vi "LabVIEW_MQTT_Toolkit_V2.vi"() -> ()   [LabVIEW 2021]
uses:
  class/mqtt/mqttTypedef/mqttQOSlevel.ctl
  class/mqtt/mqttTypedef/mqttConnectionStatus.ctl
  class/mqtt/mqttTypedef/mqttBroker.ctl
  class/mqtt/mqttTXqueue/mqttTXdataQueueFunction.ctl
  class/mqtt/mqttConfigFunction.ctl
  class/mqtt/mqttTXqueue/mqttRXsubscriptionEventFunction.ctl
  <vilib>/Utility/sysdir.llb/System Directory Type.ctl
  library/Epoch Date & Time/epoch.UNIX/Epoch.UNIX.lvclass
  C:/Users/Fujitsu/Desktop/labpublish/avril/Project mqtt/Src/library/Epoch Date & Time/epoch/Epoch.lvclass
  <vilib>/Utility/file.llb/Write Delimited Spreadsheet (string).vi
  library/Epoch Date & Time/Get Epoch Time.vi
  class/mqtt/mqtt.lvclass
panel:
  out "concatenated string":string
  in  "Tab Control":T1(tab)
  in  "Device type":u16(ring) items=["AX_3D", "AX_3DS", "HI_INC_BI", "HI_INC_MONO", "X_INC_BI", "X_INC_MONO"]
  in  "Tx ratio":u8
  in  "Store and forward":bool
  in  "Streaming options":T2(radio)
  in  "Daq options":T3(radio)=enum."Tx Only"
  out "Connection Success":bool
  in  "connect":bool
  out "ConnStatus":T4
  in  "disconnect":bool
  in  "subscribe":bool
  out "Subscribe Success":bool
  in  "Subscription_Info":cluster{"Topic":string, "QoS":T5}[](array[cluster])=[{"Topic"="MacID/Topic", "QoS"=enum."At most once"}]
  out "Subscribed_Topic":string
  out "messageID":u16
  in  "quit":bool
  in  "Broker configuration":T6={"IP or  URL of the broker"="", "connTimeout"=2000, "writeTimeout"=2000, "readTimeout"=2000, "subTimeout"=30000, "Port"=1883}
  in  "Topic":string
  out "Publish success":bool
  in  "Publish":bool
  in  "Data acq .mode":u8(ring)=1 items=["Stop"=1, "LowDutyCycle"=2, "Alarm"=4, "Streaming"=3, "S.E.T"=5, "Sock Detection"=6]
  in  "Data Acq duration":cluster{"hours":u8, "minutes":u8, " Seconds":u8} {"Seconds" max=60 format="%02.0f"; "minutes" max=60 format="%02.0f"; "hours" max=24 format="%02.0f"}
  in  "Sampling rate":u32(ring) items=["", "10 Hz", "16 Hz", "20 Hz", "25 Hz", "32 Hz", "40 Hz", "50 Hz", "64 Hz", "80 Hz", "100 Hz", "125 Hz", "160 Hz", "200 Hz", "250  Hz", "320 Hz", "400 Hz", "500 Hz", "800 Hz", "1000 Hz", "1600 Hz", "2000 Hz"]
  in  "Data acq cycle/Notif cycle":cluster{"hours":u8, "minutes":u8, " Seconds":u8} {"Seconds" max=60 format="%02.0f"; "minutes" max=60 format="%02.0f"; "hours" max=24 format="%02.0f"}
  in  "Data aging":u16=30 step=10
  in  "Mac Id":string
  in  "Math notif ratio":u16
  in  "Ping request":bool
  out "Measure Graph":dbl(graph)
  out "Measure mode":string
  out "Sensor Label":string
  out "Measure":dbl
  out "Date & time":string
  out "Device type":string
  out "End date":string
  out "Start date":string
  out "Average value":dbl
  out "Minimum value":dbl
  out "Maximum value":dbl
  out "Date":string
  out "Date":string
  out "File path":path
  out "File path":path
  out "Measure mode":string
  out "Sensor label":string
  out "Measure":dbl
  out "Date & time":string
  out "Device type":string
  out "Alarm status":string
  out "Waveform Chart":dbl(graph) caption="Measure graph"
  out "File path":path
  out "Sampling rate":i16
  out "Frame sequence Id":u32
  out "Number of daq per channel":u16
  out "Data acquisition cycle":u32
  out "Data acquisition duration":u32
  out "Prev.number of daq per channel":u16
  out "Enabled channels":string
  out "Device type":string
  out "Measure mode":string
  out "millisec":u16
  out "not synchronised":bool
  out "synchronised":bool
  out "Network quality (LQI)":u8 format="%.0p"
  out "Ref time":string
  out "INC_Y Graph":dbl[](graph)
  out "CH_Z Graph":dbl[](graph)
  out "CH_X Graph":dbl[](graph)
  out "CH_Y Graph":dbl[](graph)
  out "INC_X Graph":dbl[](graph)
  out "File path":path
  out "Enabled channels":string
  out "Device type":string
  out "Measure mode":string
  out "Frame sequence Id":u32
  out "Number of daq per channel":u16
  out "Data notification cycle":u32
  out "Data acquisition duration":u32
  out "Prev.number of daq per channel":u16
  out "not synchronised":bool
  out "synchronised":bool
  out "Network quality (LQI)":u8 format="%.0p"
  out "Sampling rate":i16
  out "millisec":u16
  out "Ref time":string
  out "channel that received alarm":u8
  out "CH_Z Graph":dbl[](graph)=[0.984, 0.974, 0.974, 0.986, 1.009, 0.965, 0.949, 0.987, 0.909, 0.979, 0.976, 1.021, 0.92, 0.95, 1.042, 0.989, 0.939, 1.09, 0.874, 0.972, 0.98, 0.977, 0.963, 0.971, 0.982, 0.977, 0.992, 0.993, 0.98, 0.969, 0.975, 0.969, 0.986, 0.985, 0.978, 0.977, 0.982, 0.979, 0.977, 0.972, 0.967, 0.968, 0.986, 0.97, 0.973, 0.977, 0.982, 0.973, 0.953, 0.969, 0.983, 0.968, 0.965, 0.975, 0.974, 0.972, 0.983, 0.99, 0.968, 0.972, 0.97, 0.981, 0.968, 0.982, 0.979, 0.972]
  out "CH_X Graph":dbl[](graph)=[0.011, 0.001, 0.002, 0.005, 0.007, 0.003, 0.001, 0.011, -0.001, 0.008, 0.006, 0.001, -0.001, 0.017, -0.002, 0.004, 0.0, -0.007, 0.002, -0.007, 0.001, 0.002, 0.0, 0.003, 0.004, 0.009, 0.004, 0.012, 0.003, 0.003, 0.004, 0.003, 0.006, 0.001, -0.001, 0.003, 0.002, 0.001, 0.003, 0.0, -0.001, 0.005, 0.0, 0.005, 0.001, 0.005, 0.005, -0.001, -0.002, -0.001, 0.005, 0.003, -0.003, -0.003, 0.002, -0.002, 0.002, 0.007, 0.0, 0.0, -0.002, 0.001, 0.002, 0.005, 0.011, 0.006]
  out "CH_Y Graph":dbl[](graph)=[-0.006, -0.012, -0.012, -0.009, -0.015, 0.009, 0.007, -0.013, 0.026, 0.009, -0.014, -0.014, 0.046, 0.055, -0.014, 0.004, 0.027, -0.027, 0.076, -0.008, -0.016, -0.026, -0.02, -0.015, -0.01, -0.002, -0.005, -0.011, -0.019, -0.019, -0.014, -0.009, -0.01, -0.01, -0.017, -0.015, -0.01, -0.013, -0.014, -0.014, -0.014, -0.014, -0.013, -0.017, -0.015, -0.013, -0.008, -0.015, -0.02, -0.017, -0.011, -0.014, -0.015, -0.016, -0.019, -0.016, -0.016, -0.012, -0.016, -0.016, -0.01, -0.013, -0.013, -0.019, -0.015, -0.012]
  out "INC_X Graph":dbl[](graph)=[0.03, 0.047, 0.036, 0.04, 0.082, 0.015, 0.021, 0.002, -0.032, 0.039, 0.026, 0.014, 0.037, 0.052, 0.099, 0.049, 0.039, 0.13, -0.382, 0.13, 0.113, 0.024, 0.006, -0.008, 0.051, 0.01, 0.082, 0.011, 0.03, 0.0, 0.031, 0.032, 0.033, 0.046, 0.032, 0.037, 0.018, 0.028, 0.024, 0.031, -0.008, 0.054, 0.011, 0.025, 0.04, 0.026, 0.022, 0.017, 0.028, 0.042, 0.024, 0.016, 0.034, 0.035, 0.018, 0.043, 0.014, 0.039, 0.033, 0.018, 0.035, 0.027, 0.041, 0.031, 0.035, 0.03]
  out "INC_Y Graph":dbl[](graph)=[0.458, 0.458, 0.458, 0.458, 0.458, 0.458, 0.458, 0.458, 0.458, 0.458, 0.458, 0.458, 0.458, 0.458, 0.458, 0.458, 0.458, 0.458, 0.458, 0.458, 0.458, 0.458, 0.458, 0.458, 0.458, 0.458, 0.458, 0.458, 0.458, 0.458, 0.458, 0.458, 0.458, 0.458, 0.458, 0.458, 0.458, 0.458, 0.458, 0.458, 0.458, 0.458, 0.458, 0.458, 0.458, 0.458, 0.458, 0.458, 0.458, 0.458, 0.458, 0.458, 0.458, 0.458, 0.458, 0.458, 0.458, 0.458, 0.458, 0.458, 0.458, 0.458, 0.458, 0.458, 0.458, 0.458]
  out "File path":path
  out "File path":path
  out "Data acquisition duration":u32
  out "Frame sequence Id":u32
  out "Data monitoring cycle":u32
  out "Device type":string
  out "Sampling rate":i16
  out "Number of daq per channel":u16
  out "Prev.number of daq per channel":u16
  out "Ref time":string
  out "millisec":u16
  out "Measure mode":string
  out "Enabled channels":string
  out "Network quality (LQI)":u8 format="%.0p"
  out "CH_Z Graph":dbl[](graph)
  out "synchronised":bool
  out "not synchronised":bool
  out "CH_Y Graph":dbl[](graph)
  out "CH_X Graph":dbl[](graph)
  out "Shock source":string
  out "Y Axis first data":dbl format="%#_5f"
  out "X Axis first data":dbl format="%#_5f"
  out "Z Axis first data":dbl format="%#_5f"
  out "Device type":string
  out "Acquisition Mode":string
  out "Acquisition frequency":u16
  out "Acquisition cycle":u32
  out "Acquisition duration":u32
  out "Enabled channels":string
  out "Start date":string
  out "End date":string
  out "Number of data per channel":u16
  out "fid min ch1":u32
  out "index minval":u16
  out "fid max ch1":u32
  out "index maxval":u16
  out "Max value":dbl[](array[numeric]) format="%#_3g"
  out "Average value":dbl[](array[numeric])
  out "Min value":dbl[](array[numeric])
  out "String":string="Ch_Z                    Ch_X                     Ch_Y                     INC_X                     INC_Y"
  out "File path":path
  out "Min date":string[](array[string])
  out "Max date":string[](array[string])
  out "Numeric":i32
  # "Publish_Info"
  # ":"
  # ":"
  # "HH:MM:SS"
  # ":"
  # ":"
  # "HH:MM:SS"
  # "LowDutyCycle Measurement"
  # "MathMode Result"
  # "AlarmMode Measurement"
  # "StreamingMode Measurement"
  # "S.E.T Mode Measurement"
  # "ShockDetectionMode Measurement"
  # "DynamicMathMode Measurement"
types:
  T1 = enum32{"Configuration", "LowDutyCycleData", "AlarmData ", "StreamingModeData", "S.E.T Mode", "Shock Detection", "Dynamic Math Result"}
  T2 = enum32{"No Selection", "Continuous Monitoring", "Burst", "One Shot"}
  T3 = enum32{"No Selection", "Tx Only", "Log Only", "Tx&Log", "SA"}
  T4 = typedef "mqttConnectionStatus.ctl" = enum16{"Connection accepted", "Connection refused: unacceptable protocol version", "Connection refused: identifier rejected", "Connection refused: Server unavailable", "Connection refused: bad user name or password", "Connection refused: not authorized"}
  T5 = typedef "mqttQOSlevel.ctl" = enum8{"At most once", "At least once", "Exactly once", "Reserved"}
  T6 = typedef "mqttBroker.ctl" = cluster{"IP or  URL of the broker":string, "connTimeout":i32, "writeTimeout":i32, "readTimeout":i32, "subTimeout":i32, "Port":u16}
  T7 = typedef "mqttRXsubscriptionEventFunction.ctl" = enum16{"init", "deinit", "getEventRef", "event"}
  T8 = typedef "mqtt.lvclass/mqttConfigFunction.ctl" = enum16{"init", "deinit", "set", "get"}
  T9 = typedef "mqttTXdataQueueFunction.ctl" = enum16{"init", "deinit", "getQueue", "enqueue"}
  T10 = enum8{"Enabled", "Disabled", "Disabled and Grayed Out"}
  T11 = enum16{"open", "replace", "create", "open or create", "replace or create", "replace or create with confirmation"}
  T12 = cluster{"[0]":u8, "[1]":u8, "[2]":u8, "[3]":u8, "[4]":u8, "[5]":u8, "[6]":u8, "[7]":u8, "[8]":u8}
  T13 = cluster{"[0]":u8, "[1]":u8, "[2]":u8, "[3]":u8, "[4]":u8, "[5]":u8, "[6]":u8, "[7]":u8, "[8]":u8, "[9]":u8, "[10]":u8, "[11]":u8, "[12]":u8}
  T14 = typedef "System Directory Type.ctl" = i32
  T15 = cluster{"unsigned byte array[0]":u8, "unsigned byte array[1]":u8}
  T16 = cluster{"[0]":u8, "[1]":u8, "[2]":u8, "[3]":u8, "[4]":u8, "[5]":u8, "[6]":u8, "[7]":u8, "[8]":u8, "[9]":u8, "[10]":u8, "[11]":u8, "[12]":u8, "[13]":u8, "[14]":u8, "[15]":u8}
  T17 = cluster{"[0]":u8, "[1]":u8, "[2]":u8, "[3]":u8, "[4]":u8, "[5]":u8, "[6]":u8, "[7]":u8, "[8]":u8, "[9]":u8, "[10]":u8, "[11]":u8, "[12]":u8, "[13]":u8, "[14]":u8, "[15]":u8, "[16]":u8, "[17]":u8, "[18]":u8, "[19]":u8, "[20]":u8, "[21]":u8}
  T18 = cluster{"unsigned byte array[0]":u8, "unsigned byte array[1]":u8, "unsigned byte array[2]":u8, "unsigned byte array[3]":u8, "unsigned byte array[4]":u8, "unsigned byte array[5]":u8, "unsigned byte array[6]":u8, "unsigned byte array[7]":u8, "unsigned byte array[8]":u8, "unsigned byte array[9]":u8, "unsigned byte array[10]":u8, "unsigned byte array[11]":u8, "unsigned byte array[12]":u8, "unsigned byte array[13]":u8, "unsigned byte array[14]":u8, "unsigned byte array[15]":u8, "unsigned byte array[16]":u8, "unsigned byte array[17]":u8, "unsigned byte array[18]":u8, "unsigned byte array[19]":u8, "unsigned byte array[20]":u8, "unsigned byte array[21]":u8, "unsigned byte array[22]":u8, "unsigned byte array[23]":u8, "unsigned byte array[24]":u8, "unsigned byte array[25]":u8, "unsigned byte array[26]":u8, "unsigned byte array[27]":u8, "unsigned byte array[28]":u8, "unsigned byte array[29]":u8, "unsigned byte array[30]":u8, "unsigned byte array[31]":u8, "unsigned byte array[32]":u8, "unsigned byte array[33]":u8, "unsigned byte array[34]":u8, "unsigned byte array[35]":u8}
  T19 = cluster{"[0]":string, "[1]":string, "[2]":string, "[3]":string, "[4]":string}
  T20 = cluster{"[0]":dbl, "[1]":dbl, "[2]":dbl, "[3]":dbl, "[4]":dbl}
diagram:
  # "here you will find different modes of  data acquisition"
  # "cluster contain broker configuration"
  n1 = flat-sequence {
    tunnel: [w20] -> w14
    tunnel: [w17] -> w9
    frame #0 {
      w16 = T10."Disabled and Grayed Out" ("Disabled")
      n2 = property on="disconnect" class="Bool"("DisabledEnum"=w16) -> ()  [unwired: 2 in, 2 out]
      n3 = property on="subscribe" class="Bool"("DisabledEnum"=w16) -> ()  [unwired: 2 in, 2 out]
      n4 = call "mqttRXsubscriptionEvent.vi"("function"=mqttRXsubscriptionEventFunction."init") -> ("subscriptionData"=w17:refnum<user-event>, "error out"=w19:errorcluster)  [unwired: 13 in]
      n5 = call "mqttTXdataQueue.vi"("function"=mqttTXdataQueueFunction."init", "error in (no error)"=w19) -> ("error out"=w20:errorcluster)  [unwired: 12 in, 1 out]
    }
  }
  n6 = register-events(w9) -> (reference out=w8:refnum<event-registration>)  [unwired: 2 in, 1 out]
  n7 = call "api_mqttInit.vi"("broker"="Broker configuration", "error in (no error)"=w14) -> ("error out"=w12:errorcluster)  [unwired: 13 in]
  n8 = call "mqttConfigStore.vi"("function"=mqttConfigFunction."get", "error in (no error)"=w12) -> ("mqtt.lvclass out"=w11:refnum<class "mqtt.lvclass">, "error out"=w1:errorcluster)  [unwired: 12 in]
  n9 = call "mqttTCPIPserver.vi"("mqtt.lvclass"=w11, "error in (no error)"=w1) -> ()  [unwired: 12 in, 2 out]
  n10 = while {
    shift-right: [w27] -> w5
    shift-left: w1 -> [w22]
    tunnel: w8 -> [w26]
    tunnel: [w25] -> w3
    i -> [w23]
    stop <- w24 stop-if-true
    n11 = event shown="[5] \"subscribe\": Value Change" {
      selector: w26 -> [_ _ _ _ _ _ _ _ _ _ _]
      dyn-events: [_ _ _ _ _ _ _ _ _ _ _] -> w25
      timeout: _ -> [_ _ _ _ _ _ _ _ _ _ _]
      tunnel: [w31 w115 w159 w162 w165 w169 w254 w6078 w6108 w6119 w6128] -> w27
      tunnel: w22 -> [w31 w116 w159 w163 w166 w167 w254 w6078 w6108 w6119 w6128]
      tunnel: [TRUE _ _ _ _ _ _ _ _ _ _] -> w24
      tunnel: w23 -> [_ _ _ _ _ _ w175 _ _ _ _]
      event "quit": Value Change {
        # "used to reinitialize to default  data when you execute VI"
        # "when we press quit in front panel the process is stopped"
        n12 = event-data() -> ()  [unwired: 1 in, 1 out]
        n13 = control-ref of="This VI"() -> (w30:refnum<vi>)
        n14 = invoke class="VI" method="Default Vals.Reinit All"(reference=w30) -> (reference out=w28:refnum<vi>, error out=w29:errorcluster)  [unwired: 2 in, 1 out]
        n15 = Close Reference(reference=w28, error in (no error)=w29) -> ()  [unwired: 1 out]
      }
      event "Publish": Value Change {
        w37 = u8 0
        w38 = u8 0
        w52 = u8 16
        w53 = u8 23
        # "publish button"
        # "this is math constant \"3600\" to stop the process"
        n16 = event-data() -> ()  [unwired: 1 in, 1 out]
        n17 = String Subset(string="Mac Id", length (rest)=15 ("length (rest)")) -> (substring=w112:string)  [unwired: 1 in]
        n18 = String Length(string=w112) -> (length=w113:i32)
        n19 = call <vilib>:"Trim Whitespace.vi"("string"=w112) -> ("trimmed string"=w111:string)  [unwired: 1 in]
        n20 = for {
          N: w113 -> [_]
          tunnel: w111 -> [w158]
          tunnel: [w155] -> w110 mode=indexing
          i -> [w154]
          n21 = Multiply(x=w154, y=2) -> (x*y=w152:i32)
          n22 = String Subset(string=w158, offset (0)=w152, length (rest)=2 ("length (rest)")) -> (substring=w156:string)
          n23 = Hexadecimal String To Number(string=w156) -> (number=w155:u32)  [unwired: 2 in, 1 out]
        }
        n24 = Unbundle By Name("Data acq cycle/Notif cycle") -> ("hours"=w85:u8, "minutes"=w84:u8, "Seconds"=w83:u8)
        n25 = Unbundle By Name("Data Acq duration") -> ("hours"=w74:u8, "minutes"=w73:u8, "Seconds"=w72:u8)
        n26 = Multiply(x=w83, y=1.0) -> (x*y=w92:dbl)
        n27 = Multiply(x=w72, y=1.0) -> (x*y=w79:dbl)
        n28 = Multiply(x=w84, y=60.0) -> (x*y=w91:dbl)
        n29 = Multiply(x=w73, y=60.0) -> (x*y=w78:dbl)
        n30 = Multiply(x=w85, y=3600.0) -> (x*y=w90:dbl)
        n31 = case shown="0, Default" "Sampling rate" {
          tunnel: [10 16 20 25 32 40 50 64 80 100 125 160 200 250 320 400 500 800 1000 1600 0 2000] -> w39
          frame 1 {
          }
          frame 2 {
          }
          frame 3 {
          }
          frame 4 {
          }
          frame 5 {
          }
          frame 6 {
          }
          frame 7 {
          }
          frame 8 {
          }
          frame 9 {
          }
          frame 10 {
          }
          frame 11 {
          }
          frame 12 {
          }
          frame 13 {
          }
          frame 14 {
          }
          frame 15 {
          }
          frame 16 {
          }
          frame 17 {
          }
          frame 18 {
          }
          frame 19 {
          }
          frame 20 {
          }
          frame 0, Default {
          }
          frame 21 {
          }
        }
        n32 = property on="Streaming options" class="RadioBtnsControl (strict)"() -> ("Value"=w44:T2)  [unwired: 2 in, 2 out]
        n33 = Add(x=w92, y=w91) -> (x+y=w89:dbl)
        n34 = Add(x=w79, y=w78) -> (x+y=w76:dbl)
        n35 = Multiply(x=w74, y=3600.0) -> (x*y=w77:dbl)
        n36 = case shown="True" "Store and forward" {
          tunnel: [u16 0 "Data aging"] -> w59
          frame False {
          }
          frame True {
          }
        }
        n37 = Add(x=w89, y=w90) -> (x+y=w71:dbl)
        n38 = Add(x=w76, y=w77) -> (x+y=w68:dbl)
        n39 = case shown="\"Tx Only\"" "Daq options" {
          tunnel: [u8 32 u8 1 u8 0 u8 33 u8 64] -> w106
          frame "Tx Only" {
          }
          frame "Log Only" {
          }
          frame "No Selection", Default {
          }
          frame "Tx&Log" {
          }
          frame "SA" {
          }
        }
        n40 = case shown="\"Continuous Monitoring\"" w44 {
          tunnel: [u8 0 ("index") u8 4 u8 12 u8 8] -> w105
          frame "No Selection", Default {
          }
          frame "Continuous Monitoring" {
          }
          frame "Burst" {
          }
          frame "One Shot" {
          }
        }
        n41 = To Unsigned Long Integer(number=w71) -> (unsigned 32bit integer=w102:u32)
        n42 = To Unsigned Long Integer(number=w68) -> (unsigned 32bit integer=w70:u32)
        n43 = To Unsigned Byte Integer(number=w110) -> (unsigned 8bit integer=w88:u8[])
        n44 = Split Number(x=w39) -> (hi(x)=w63:u16, lo(x)=w62:u16)
        n45 = Split Number(x=w102) -> (hi(x)=w100:u16, lo(x)=w101:u16)
        n46 = Split Number(x=w70) -> (hi(x)=w69:u16, lo(x)=w67:u16)
        n47 = Add(x=w106, y=w105) -> (x+y=w51:u8)
        n48 = Split Number(x=w63) -> (lo(x)=w60:u8)  [unwired: 1 out]
        n49 = Split Number(x=w100) -> (lo(x)=w96:u8)  [unwired: 1 out]
        n50 = Split Number(x=w69) -> (lo(x)=w64:u8)  [unwired: 1 out]
        n51 = Split Number(x=w62) -> (hi(x)=w56:u8, lo(x)=w61:u8)
        n52 = Split Number(x=w59) -> (hi(x)=w57:u8, lo(x)=w58:u8)
        n53 = Split Number(x="Math notif ratio") -> (hi(x)=w35:u8, lo(x)=w34:u8)
        n54 = Split Number(x=w101) -> (hi(x)=w97:u8, lo(x)=w98:u8)
        n55 = Split Number(x=w67) -> (hi(x)=w65:u8, lo(x)=w66:u8)
        n56 = Array Subset(array=w88, index=0, length=8) -> (w54:u8[])
        n57 = Build Array (concatenate)(w54, w53, w52, "Data acq .mode", w51, u8 0, u8 0, u8 0, w98, w97, w96, "Tx ratio", w66, w65, w64, w61, w56, w60, w38, w38, w38, w58, w57, w34, w35) -> (w46:u8[])
        n58 = Build Array (concatenate)(w54, w53, w52, "Data acq .mode", w51, w37, w37, w37, w37, w37, w37, "Tx ratio", w37, w37, w37, w37, w37, w37, w37, w37, w37, w37, w37, u8 16, u8 14) -> (w47:u8[])
        n59 = Equal?(x="Data acq .mode", y=u8 1) -> (x = y?=w48:bool)
        n60 = Select(t=w47, s=w48, f=w46) -> (s? t:f=w45:u8[])
        n61 = call "api_mqttPublish.vi"("topic"="Topic", "value"=w45, "QoS (At most once)"=mqttQOSlevel."At most once", "error in (no error)"=w116) -> ("success"=→"Publish success":bool, "error out"=w115:errorcluster)  [unwired: 10 in]
      }
      event "Ping request": Value Change {
        n62 = event-data() -> ()  [unwired: 1 in, 1 out]
        n63 = call "api_mqttPing.vi"("error in (no error)"=w159) -> ()  [unwired: 13 in, 2 out]
      }
      event "connect": Value Change {
        # "when the connection is accepted subscribe+disconnect become enabled"
        # "this button is to conect to the broker"
        n64 = event-data() -> ()  [unwired: 1 in, 4 out]
        n65 = call "api_mqttConnect.vi"("error in (no error)"=w163) -> ("success"=→"Connection Success":bool, "connStatus"=w161:T4, "error out"=w162:errorcluster)  [unwired: 11 in, 1 out]
        "ConnStatus" <- w161
        n66 = case shown="\"Connection accepted\"" w161 {
          frame "Connection accepted" {
            w164 = T10."Enabled" ("Disabled")
            n67 = property on="disconnect" class="Bool"("DisabledEnum"=w164) -> ()  [unwired: 2 in, 2 out]
            n68 = property on="subscribe" class="Bool"("DisabledEnum"=w164) -> ()  [unwired: 2 in, 2 out]
          }
          frame Default {
          }
        }
      }
      event "disconnect": Value Change {
        n69 = event-data() -> ()  [unwired: 1 in, 4 out]
        n70 = call "api_mqttDisconnect.vi"("error in (no error)"=w166) -> ("error out"=w165:errorcluster)  [unwired: 13 in, 1 out]
      }
      event "subscribe": Value Change {
        # "contain topic to which we will subscribe"
        # "this indicator turn to green when the subscription sucssed"
        n71 = event-data() -> ()  [unwired: 1 in, 4 out]
        n72 = feedback #1(u16 0) -> (w172:u16)
        n73 = Increment(x=w172) -> (x+1=w168:u16)
        n74 = feedback-in #1(w168) -> ()
        n75 = call "api_mqttSubscribe.vi"("subscriptionInfo"="Subscription_Info", "messageID"=w168, "error in (no error)"=w167) -> ("success"=→"Subscribe Success":bool, "error out"=w169:errorcluster)  [unwired: 11 in]
      }
      event User Event {
        n76 = event-data() -> ("topic"=w174:string, "value"=w188:string, "messageID"=→"messageID":u16)  [unwired: 1 in]
        "Subscribed_Topic" <- w174
        n77 = String To Byte Array(string=w188) -> (unsigned byte array=w196:u8[])
        n78 = Reverse 1D Array(array=w196) -> (reversed array=w240:u8[])
        n79 = Array Subset(array=w196, index=0, length=7) -> (w191:u8[])
        n80 = Array Subset(array=w196, index=7, length=1) -> (w198:u8[])
        n81 = Array Subset(array=w196, index=3, length=13) -> (w233:u8[])
        n82 = Array To Cluster(array=w191) -> (cluster=w246:T12)
        n83 = Array To Cluster(array=w198) -> (cluster=w197:cluster{"[0]":u8})
        n84 = Array To Cluster(array=w233) -> (cluster=w232:T13)
        n85 = Array Subset(array=w240, index=0, length=3) -> (w179:u8[])
        n86 = Unbundle By Name(w197) -> ("[0]"=w177:u8)
        n87 = Unbundle By Name(w232) -> ("[0]"=w189:u8, "[1]"=w212:u8, "[2]"=w211:u8, "[3]"=w210:u8, "[4]"=w209:u8, "[5]"=w216:u8, "[6]"=w215:u8, "[7]"=w214:u8, "[8]"=w213:u8, "[9]"=w206:u8, "[10]"=w205:u8, "[11]"=w208:u8, "[12]"=w207:u8)
        n88 = Unbundle By Name(w246) -> ("[0]"=w178:u8, "[1]"=w204:u8, "[2]"=w241:u8, "[3]"=w245:u8, "[4]"=w244:u8, "[5]"=w243:u8, "[6]"=w242:u8)
        n89 = Array To Cluster(array=w179) -> (cluster=w186:cluster{"[0]":u8, "[1]":u8, "[2]":u8})
        n90 = Join Numbers(hi=w244, lo=w245) -> ((hi.lo)=w236:u16)
        n91 = Join Numbers(hi=w242, lo=w243) -> ((hi.lo)=w237:u16)
        n92 = Join Numbers(hi=w211, lo=w212) -> ((hi.lo)=w227:u16)
        n93 = Join Numbers(hi=w209, lo=w210) -> ((hi.lo)=w228:u16)
        n94 = Join Numbers(hi=w215, lo=w216) -> ((hi.lo)=w222:u16)
        n95 = Join Numbers(hi=w213, lo=w214) -> ((hi.lo)=w223:u16)
        n96 = Join Numbers(hi=w205, lo=w206) -> ((hi.lo)=w217:u16)
        n97 = Join Numbers(hi=w207, lo=w208) -> ((hi.lo)=w218:u16)
        n98 = case shown="1" w178 {
          tunnel: ["AX-3D" "HI_INC_MONO" "HI_INC_BI" "X_INC_MONO " "X _INC_BI " "AX_3DS" ""] -> w187
          frame 1 {
          }
          frame 2 {
          }
          frame 3 {
          }
          frame 4 {
          }
          frame 5 {
          }
          frame 6 {
          }
          frame Default {
          }
        }
        "Device type" <- w187
        n99 = case shown="1" w241 {
          tunnel: ["Ch_Z" "Ch_Y" "INC_X" "INC_Y" "" "Ch_X"] -> w176
          frame 0 {
          }
          frame 2 {
          }
          frame 3 {
          }
          frame 4 {
          }
          frame Default {
          }
          frame 1 {
          }
        }
        n100 = Unbundle(w186) -> ("[0]"=w183:u8, "[1]"=w184:u8, "[2]"=w185:u8)
        n101 = Join Numbers(hi=w184, lo=w185) -> ((hi.lo)=w181:u16)
        n102 = To Unsigned Word Integer(number=w236) -> (unsigned 16bit integer=w249:u16)
        n103 = To Unsigned Word Integer(number=w237) -> (unsigned 16bit integer=w250:u16)
        n104 = To Unsigned Word Integer(number=w227) -> (unsigned 16bit integer=w229:u16)
        n105 = To Unsigned Word Integer(number=w228) -> (unsigned 16bit integer=w230:u16)
        n106 = To Unsigned Word Integer(number=w222) -> (unsigned 16bit integer=w224:u16)
        n107 = To Unsigned Word Integer(number=w223) -> (unsigned 16bit integer=w225:u16)
        n108 = To Unsigned Word Integer(number=w217) -> (unsigned 16bit integer=w219:u16)
        n109 = To Unsigned Word Integer(number=w218) -> (unsigned 16bit integer=w220:u16)
        n110 = Join Numbers(hi=w250, lo=w249) -> ((hi.lo)=w251:u32)
        n111 = Join Numbers(hi=w230, lo=w229) -> ((hi.lo)=w231:u32)
        n112 = Join Numbers(hi=w225, lo=w224) -> ((hi.lo)=w226:u32)
        n113 = Join Numbers(hi=w220, lo=w219) -> ((hi.lo)=w221:u32)
        n114 = To Word Integer(number=w183) -> (16bit integer=w252:i16)
        n115 = Sign(1:w252) -> (0:w182:i16)
        n116 = To Unsigned Long Integer(number=w251) -> (unsigned 32bit integer=w203:u32)
        n117 = To Unsigned Long Integer(number=w231) -> (unsigned 32bit integer=w200:u32)
        n118 = To Unsigned Long Integer(number=w226) -> (unsigned 32bit integer=w201:u32)
        n119 = To Unsigned Long Integer(number=w221) -> (unsigned 32bit integer=w202:u32)
        n120 = case shown="6" w204 {
          tunnel: ["" w300 w338 "Streaming mode" "Shock Detection" "LDC Math Result" "S.E.T mode " "Dynamic Math Result"] -> w195
          tunnel: w203 -> [_ w306 w363 _ _ _ _ _]
          tunnel: [_ w265 w319 _ _ "" _ _] -> w190
          tunnel: w187 -> [w261 w302 w339 w538 w2873 w3420 w3588 w5910]
          tunnel: [w261 w302 w339 w538 w2873 w3420 w3588 w5910] -> w194
          tunnel: w176 -> [_ w299 w329 w537 w2872 w3418 _ w5909]
          tunnel: [_ w299 w329 w537 w2872 w3418 _ w5909] -> w193
          tunnel: w182 -> [_ w308 w361 _ _ w3414 _ _]
          tunnel: w181 -> [_ w307 w362 _ _ w3416 _ _]
          tunnel: [_ w303 w337 _ _ _ _ _] -> w180
          tunnel: w189 -> [_ _ _ _ _ w3415 _ _]
          tunnel: w202 -> [_ _ _ _ _ w3417 _ _]
          tunnel: w201 -> [_ _ _ _ _ w3372 _ _]
          tunnel: w200 -> [_ _ _ _ _ w3373 _ _]
          tunnel: w188 -> [_ _ _ w484 w2819 _ w3577 w5907]
          tunnel: w187 -> [_ _ _ _ _ _ _ w5908]
          tunnel: w179 -> [_ _ _ _ _ _ _ _]
          tunnel: w174 -> [_ _ _ w387 w2731 w3378 _ _]
          tunnel: w174 -> [_ _ w324 _ _ _ w3443 w5755]
          tunnel: w174 -> [_ w271 _ _ _ _ _ _]
          tunnel: w178 -> [_ _ _ _ _ _ _ w5793]
          tunnel: w177 -> [_ _ w332 _ _ _ _ _]
          tunnel: w176 -> [_ w274 _ _ _ w3383 _ _]
          frame Default {
          }
          frame 1 {
            w281 = T14 2 items=["User Home"=0, "User Desktop"=1, "User Documents"=2, "User Application Data"=3, "User Preferences"=4, "User Temporary"=5, "Public Documents"=6, "Public Application Data"=7, "Public Preferences"=8, "Public Cache"=13, "System Core Libraries"=9, "System Installed Libraries"=10, "Application Files"=11, "Boot Volume Root"=12] ("system directory type")
            w300 = "LDCDA mode"
            # "this function show time of every value measured"
            # "function to display measures for lowduty cycle"
            # "function to write data in log file"
            # "in this block we convert data to double + sign"
            n121 = call <vilib>:"Get System Directory.vi"("system directory type"=w281) -> ("system directory"=w287:path)  [unwired: 10 in]
            n122 = Build Path(base path=w287, name or relative path="Logfile") -> (appended path=w288:path)
            n123 = call <vilib>:"Check if File or Folder Exists.vi"("path"=w288) -> ("file or folder exists?"=w289:bool, "dup path"=w290:path)  [unwired: 8 in, 1 out]
            n124 = case shown="0" w308 {
              tunnel: [_ w313 w316] -> w303
              tunnel: w307 -> [_ w312 w315]
              frame Default {
              }
              frame 1 {
                n125 = Divide(x=w312, y=-1000.0) -> (x/y=w313:dbl)
              }
              frame 0 {
                n126 = Divide(x=w315, y=1000.0) -> (x/y=w316:dbl)
              }
            }
            "Measure Graph" <- w303
            n127 = call "Unix Time to Timestamp.vi"("Unix Time (s)"=w306) -> ("Timestamp"=w305:timestamp)  [unwired: 9 in, 1 out]
            n128 = String Subset(string=w271, offset (0)=0, length (rest)=16 ("length (rest)")) -> (substring=w268:string)
            n129 = case shown="False" w289 {
              tunnel: w290 -> [w310 w311]
              tunnel: [w309 w311] -> w291
              frame False {
                n130 = Create Folder(path (use dialog)=w310) -> (created path=w309:path)  [unwired: 2 in, 2 out]
              }
              frame True {
              }
            }
            n131 = Concatenate Strings "Concatenate Strings"(w268, "_" ("string"), w274, "_" ("string"), "transmit_LowDutyCycle.csv") -> (w293:string)
            n132 = Number To Fractional String(number=w303, precision (6)=i16 3) -> (F-format string=w301:string)  [unwired: 2 in]
            n133 = Format Date/Time String(seconds (now)=w305, UTC format=TRUE) -> (date/time string=w265:string)  [unwired: 1 in]
            n134 = Build Array(w302, w300, w299, w265, w301) -> (w295:string[])
            n135 = Build Path(base path=w291, name or relative path=w293) -> (appended path=w292:path)
            n136 = Scan From String(format string="%<%x %H:%M:%S>T", input string=w265) -> (output 1=w264:timestamp)  [unwired: 3 in, 3 out]
            n137 = To Double Precision Float(number=w264) -> (double precision float=w263:dbl)
            n138 = Open/Create/Replace File(file path (use dialog)=w292, operation (0:open)=T11."open or create") -> (refnum out=w283:refnum<file>, error out=w285:errorcluster)  [unwired: 4 in, 1 out]
            n139 = Concatenate Strings("Device Type ;Measure mode;Sensor label;date & time;Measure  ", "\n") -> (w282:string)
            n140 = Write to Text File(file (use dialog)=w283, text=w282, error in=w285) -> (refnum out=w284:refnum<file>, error out=w286:errorcluster)  [unwired: 1 in, 1 out]
            n141 = property on="Measure Graph" class="WFChart (strict)"("XScale.Offset"=w263) -> ()  [unwired: 2 in, 2 out]
            n142 = Close File(refnum=w284, error in=w286) -> (path=w276:path)  [unwired: 1 out]
            "File path" <- w276
            n143 = call-poly <vilib>:"Write Delimited Spreadsheet.vi"("file path (dialog if empty)"=w276, "format (%s)"="%s" ("format (%.3f)"), "1D data"=w295, "append to file? (new file:F)"=TRUE, "transpose? (no:F)"=FALSE, "delimiter (\\t)"=";" ("delimiter (\\t)")) -> ()  [unwired: 8 in, 2 out]
          }
          frame 2 {
            w347 = T14 2 items=["User Home"=0, "User Desktop"=1, "User Documents"=2, "User Application Data"=3, "User Preferences"=4, "User Temporary"=5, "Public Documents"=6, "Public Application Data"=7, "Public Preferences"=8, "Public Cache"=13, "System Core Libraries"=9, "System Installed Libraries"=10, "Application Files"=11, "Boot Volume Root"=12] ("system directory type")
            w338 = "Alarm mode"
            # "date/time string is in Universal Time"
            # "function to write measures in logfile"
            # "function to set time of measure as an offset"
            # "function to display measures in graph"
            # "this block contain different alarm status"
            # "in this block we convert data to double + sign"
            n144 = case shown="1" w361 {
              tunnel: [_ w377 w380] -> w337
              tunnel: w362 -> [_ w376 w379]
              frame Default {
              }
              frame 1 {
                n145 = Divide(x=w376, y=-1000.0) -> (x/y=w377:dbl)
              }
              frame 0 {
                n146 = Divide(x=w379, y=1000.0) -> (x/y=w380:dbl)
              }
            }
            "Waveform Chart" <- w337
            n147 = String Subset(string=w324, offset (0)=0, length (rest)=16 ("length (rest)")) -> (substring=w323:string)
            n148 = case shown="0" w332 {
              tunnel: ["" "No Alert         " "Alert Start   " "Alert  in progress" "Alert  End   " "Action Start" "Action in Progress" "Alarm Start" "Alarm Progress"] -> w331
              frame Default {
              }
              frame 0 {
              }
              frame 1 {
              }
              frame 2 {
              }
              frame 3 {
              }
              frame 4 {
              }
              frame 5 {
              }
              frame 6 {
              }
              frame 7 {
              }
            }
            "Alarm status" <- w331
            n149 = call <vilib>:"Get System Directory.vi"("system directory type"=w347) -> ("system directory"=w348:path)  [unwired: 10 in]
            n150 = Concatenate Strings(w323, "_" ("string"), w329, "_" ("string"), "Transmit_AlarmMode.csv") -> (w340:string)
            n151 = Build Path(base path=w348, name or relative path="Logfile") -> (appended path=w345:path)
            n152 = call <vilib>:"Check if File or Folder Exists.vi"("path"=w345) -> ("file or folder exists?"=w344:bool, "dup path"=w343:path)  [unwired: 8 in, 1 out]
            n153 = case shown="False" w344 {
              tunnel: w343 -> [w374 w375]
              tunnel: [w373 w375] -> w342
              frame False {
                n154 = Create Folder(path (use dialog)=w374) -> (created path=w373:path)  [unwired: 2 in, 2 out]
              }
              frame True {
              }
            }
            n155 = call "Unix Time to Timestamp.vi"("Unix Time (s)"=w363) -> ("Timestamp"=w360:timestamp)  [unwired: 9 in, 1 out]
            n156 = Format Date/Time String(seconds (now)=w360, UTC format=TRUE) -> (date/time string=w319:string)  [unwired: 1 in]
            n157 = Build Path(base path=w342, name or relative path=w340) -> (appended path=w341:path)
            n158 = Format Into String(format string="%s;%s;%s;%s;%s;%.3f", w339, w338, w329, w319, w331, w337) -> (resulting string=w333:string)  [unwired: 2 in, 1 out]
            n159 = Scan From String(format string="%<%x %H:%M:%S>T", input string=w319) -> (output 1=w320:timestamp)  [unwired: 3 in, 3 out]
            n160 = To Double Precision Float(number=w320) -> (double precision float=w318:dbl)
            n161 = Build Array(w333) -> (w335:string[])
            n162 = property on="Waveform Chart" class="WFChart (strict)"("XScale.Offset"=w318) -> ()  [unwired: 2 in, 2 out]
            n163 = Open/Create/Replace File(file path (use dialog)=w341, operation (0:open)=T11."open or create") -> (refnum out=w355:refnum<file>, error out=w353:errorcluster)  [unwired: 4 in, 1 out]
            n164 = Concatenate Strings("Device Type ;Measure mode;Sensor label;date & time;Alarm status ;Measure  ", "\n") -> (w356:string)
            n165 = Write to Text File(file (use dialog)=w355, text=w356, error in=w353) -> (refnum out=w354:refnum<file>, error out=w352:errorcluster)  [unwired: 1 in, 1 out]
            n166 = Close File(refnum=w354, error in=w352) -> (path=w334:path)  [unwired: 1 out]
            "File path" <- w334
            n167 = call-poly <vilib>:"Write Delimited Spreadsheet.vi"("file path (dialog if empty)"=w334, "1D data"=w335, "append to file? (new file:F)"=TRUE, "transpose? (no:F)"=TRUE, "delimiter (\\t)"=";") -> ()  [unwired: 9 in, 2 out]
          }
          frame 3 {
            # "this block contain measures+ time stamp which saved in the logfile"
            # "this block contain measured values"
            # "this block contain different device type"
            # "function towrite headers of the logfile"
            # "this block contain different types of streaming mode"
            # "function to calculate timestamp"
            n168 = String Subset(string=w387, offset (0)=0, length (rest)=16 ("length (rest)")) -> (substring=w386:string)
            n169 = String To Byte Array(string=w484) -> (unsigned byte array=w494:u8[])
            n170 = Array Size(array=w494) -> (size(s)=w495:i32)
            n171 = Array To Cluster(array=w494) -> (cluster=w503:T15)
            n172 = Array Subset(array=w494, index=10, length=4) -> (w530:u8[])
            n173 = Array Subset(array=w494, index=14, length=15) -> (w525:u8[])
            n174 = Unbundle(w503) -> ("unsigned byte array[0]"=w461:u8, "unsigned byte array[1]"=w502:u8)
            n175 = Array To Cluster(array=w530) -> (cluster=w529:T12)
            n176 = Array To Cluster(array=w525) -> (cluster=w524:T16)
            n177 = Array Subset(array=w494, index=2, length=8) -> (w534:u8[])
            n178 = Subtract(x=w495, y=29) -> (x-y=w490:i32)
            n179 = Unbundle By Name(w529) -> ("[0]"=w528:u8)
            n180 = Array To Cluster(array=w534) -> (cluster=w533:T12)
            n181 = Unbundle By Name(w524) -> ("[0]"=w523:u8, "[1]"=w385:u8, "[2]"=w522:u8, "[3]"=w519:u8, "[4]"=w518:u8, "[5]"=w516:u8, "[6]"=w515:u8, "[7]"=w514:u8, "[8]"=w511:u8, "[9]"=w510:u8, "[10]"=w509:u8, "[11]"=w506:u8, "[12]"=w505:u8, "[13]"=w499:u8, "[14]"=→"Network quality (LQI)":u8)
            n182 = Array Subset(array=w494, index=29, length=w490) -> (w492:u8[])
            n183 = Unbundle By Name(w533) -> ("[0]"=w475:u8, "[1]"=w476:u8, "[2]"=w479:u8, "[3]"=w480:u8, "[4]"=w473:u8, "[5]"=w474:u8, "[6]"=w482:u8, "[7]"=w481:u8)
            n184 = Join Numbers "time"(hi=w476, lo=w475) -> ((hi.lo)=w472:u16)
            n185 = Join Numbers "date"(hi=w480, lo=w479) -> ((hi.lo)=w478:u16)
            n186 = Join Numbers(hi=w518, lo=w519) -> ((hi.lo)=w517:u16)
            n187 = Join Numbers(hi=w385, lo=w523) -> ((hi.lo)=w521:u16)
            n188 = Join Numbers(hi=w481, lo=w482) -> ((hi.lo)=w483:u16)
            n189 = Join Numbers(hi=w505, lo=w506) -> ((hi.lo)=w504:u16)
            n190 = Join Numbers(hi=w515, lo=w516) -> ((hi.lo)=w513:u16)
            n191 = Join Numbers(hi=w510, lo=w511) -> ((hi.lo)=w508:u16)
            n192 = Equal To 0?(x=w499) -> (x = 0?=→"not synchronised":bool)
            n193 = Not Equal To 0?(x=w499) -> (x != 0?=→"synchronised":bool)
            n194 = Join Numbers(hi=w474, lo=w473) -> ((hi.lo)=w465:u16)
            "millisec" <- w465
            n195 = Decimate 1D Array(w492) -> (w485:u8[], w491:u8[], w489:u8[])
            n196 = Join Numbers(hi=w522, lo=w521) -> ((hi.lo)=w520:u32)
            n197 = Join Numbers(hi=w491, lo=w485) -> ((hi.lo)=w488:u16[])
            n198 = Join Numbers(hi=w514, lo=w513) -> ((hi.lo)=w512:u32)
            n199 = Join Numbers(hi=w509, lo=w508) -> ((hi.lo)=w507:u32)
            n200 = To Word Integer(number=w504) -> (16bit integer=→"Prev.number of daq per channel":i16)
            n201 = To Word Integer(number=w517) -> (16bit integer=w486:i16)
            "Number of daq per channel" <- w486
            n202 = To Long Integer(number=w520) -> (32bit integer=w487:i32)
            "Frame sequence Id" <- w487
            n203 = To Long Integer(number=w512) -> (32bit integer=w407:i32)
            "Data acquisition cycle" <- w407
            n204 = To Long Integer(number=w507) -> (32bit integer=w408:i32)
            "Data acquisition duration" <- w408
            n205 = Divide(x=w465, y=i16 1000) -> (x/y=w466:dbl)
            n206 = for {
              tunnel: w489 -> [w2647] mode=indexing
              tunnel: [w2645] -> w440 mode=indexing
              tunnel: w488 -> [w2643] mode=indexing
              n207 = To Word Integer(number=w2647) -> (16bit integer=w2644:i16)
              n208 = Sign(1:w2644) -> (0:w2646:i16)
              n209 = case shown="1" w2646 {
                tunnel: [_ w2649 w2652] -> w2645
                tunnel: w2643 -> [_ w2648 w2651]
                frame Default {
                }
                frame 1 {
                  n210 = Divide(x=w2648, y=-1000.0) -> (x/y=w2649:dbl)
                }
                frame 0 {
                  n211 = Divide(x=w2651, y=1000.0) -> (x/y=w2652:dbl)
                }
              }
            }
            n212 = To Unsigned Word Integer(number=w466) -> (unsigned 16bit integer=w470:u16)
            n213 = case shown="4" w502 {
              tunnel: ["" "LDCDA mode" "Alarm mode" "Streaming mode" "Shock Detection mode" "LDC Math Result" "SET mode " "Dynamic Math Result"] -> w435
              tunnel: w408 -> [_ _ _ w2662 _ _ _ _]
              tunnel: w407 -> [_ _ _ w2674 _ _ _ _]
              tunnel: [w2654 _ _ w2665 _ _ _ _] -> w433
              tunnel: [w2654 _ _ w2659 _ _ _ _] -> w432
              tunnel: [w2654 _ _ w2658 _ _ _ _] -> w431
              frame Default {
                w2654 = ""
              }
              frame 1 {
              }
              frame 2 {
              }
              frame 3 {
                n214 = Equal To 0?(x=w2674) -> (x = 0?=w2676:bool)
                n215 = Greater Than 0?(x=w2674) -> (x > 0?=w2660:bool)
                n216 = Equal To 0?(x=w2674) -> (x = 0?=w2672:bool)
                n217 = Equal To 0?(x=w2662) -> (x = 0?=w2673:bool)
                n218 = Greater Than 0?(x=w2662) -> (x > 0?=w2661:bool)
                n219 = And(x=w2676, y=w2661) -> (x .and. y?=w2670:bool)
                n220 = And(x=w2661, y=w2660) -> (x .and. y?=w2669:bool)
                n221 = And(x=w2673, y=w2672) -> (x .and. y?=w2671:bool)
                n222 = Select(t="burst", s=w2669, f="") -> (s? t:f=w2659:string)
                n223 = Select(t="one shot", s=w2670, f="") -> (s? t:f=w2665:string)
                n224 = Select(t="continuous monitoring", s=w2671, f="") -> (s? t:f=w2658:string)
              }
              frame 4 {
              }
              frame 5 {
              }
              frame 6 {
              }
              frame 7 {
              }
            }
            n225 = Multiply(x=w486, y=w487) -> (x*y=w459:i32)
            n226 = Add(x=w472, y=w470) -> (x+y=w439:u16)
            n227 = To Unsigned Word Integer(number=w478) -> (unsigned 16bit integer=w438:u16)
            n228 = Join Numbers(hi=w438, lo=w439) -> ((hi.lo)=w477:u32)
            n229 = To Unsigned Quad Integer(1:w459) -> (0:w458:u64)
            n230 = Increment(x=w458) -> (x+1=w462:u64)
            n231 = To Unsigned Quad Integer(1:w477) -> (0:w471:u64)
            n232 = for {
              N: w462 -> [_]
              tunnel: w458 -> [w2642]
              tunnel: [w2642] -> w464
            }
            n233 = call "Unix Time to Timestamp.vi"("Fractional Second"=w466, "Unix Time (s)"=w471) -> ("Timestamp"=w468:timestamp)  [unwired: 8 in, 1 out]
            n234 = To Unsigned Byte Integer(number=w528) -> (unsigned 8bit integer=w442:u8)
            n235 = Format Date/Time String(time format string (%c)="%x %X %3u", seconds (now)=w468, UTC format=TRUE) -> (date/time string=w401:string)
            "Ref time" <- w401
            n236 = Decrement(x=w464) -> (x-1=w463:u64)
            n237 = for {
              tunnel: w440 -> [w2641] mode=indexing
              shift-right: [w2639] -> _
              shift-left: w463 -> [w2640]
              tunnel: [w2638] -> w460 mode=indexing
              tunnel: [w2641] -> _ mode=indexing
              n238 = Increment(x=w2640) -> (x+1=w2639:u64)
              n239 = To Unsigned Quad Integer(1:w2639) -> (0:w2638:u64)
            }
            n240 = case shown="6" w461 {
              tunnel: ["AX-3D" "HI_INC_MONO" "HI_INC_BI" "X_INC_MONO " "X _INC_BI " "AX_3DS" ""] -> w384
              frame 1 {
              }
              frame 2 {
              }
              frame 3 {
              }
              frame 4 {
              }
              frame 5 {
              }
              frame 6 {
              }
              frame Default {
              }
            }
            "Device type" <- w384
            n241 = Search and Replace String(replace all?=TRUE ("replace all? (F)"), input string=w401, search string=":", replace string="_") -> (result string=w422:string)  [unwired: 4 in, 3 out]
            n242 = To Word Integer(number=w483) -> (16bit integer=w409:i16)
            "Sampling rate" <- w409
            n243 = Search and Replace String(replace all?=TRUE ("replace all? (F)"), input string=w422, search string=",", replace string="_") -> (result string=w421:string)  [unwired: 4 in, 3 out]
            n244 = call <vilib>:"Space Constant.vi"() -> ("String"=w434:string)
            n245 = Concatenate Strings(w435, w434, w433, w432, w431) -> (w382:string)
            "Measure mode" <- w382
            "concatenated string" <- w382
            n246 = Search and Replace String(replace all?=TRUE ("replace all? (F)"), input string=w421, search string="/", replace string="_") -> (result string=w417:string)  [unwired: 4 in, 3 out]
            n247 = Number To Decimal String(number=w409) -> (decimal integer string=w398:string)  [unwired: 1 in]
            n248 = Number To Decimal String(number=w407) -> (decimal integer string=w395:string)  [unwired: 1 in]
            n249 = Number To Decimal String(number=w408) -> (decimal integer string=w392:string)  [unwired: 1 in]
            n250 = String Subset(string=w417, offset (0)=0, length (rest)=20 ("length (rest)")) -> (substring=w414:string)
            n251 = Concatenate Strings("Device type :", w384, ";", "Measure Mode :", w382, ";", "Time reference :" ("string"), w401, ";", " Sampling rate :", w398, ";" ("string"), "Data acquisition cycle :" ("string"), w395, ";" ("string"), "Data acquisition duration :" ("string"), w392, ";" ("string"), "\n") -> (w411:string)
            n252 = call <vilib>:"Space Constant.vi"() -> ("String"=w413:string)
            n253 = To Double Precision Float(number=w409) -> (double precision float=w436:dbl)
            n254 = Build Array(w411) -> (w406:string[])
            n255 = To Unsigned Quad Integer(1:w460) -> (0:w437:u64[])
            n256 = Concatenate Strings(w414, "_" ("string"), w386, w413) -> (w427:string)
            n257 = case shown="1101" w442 {
              tunnel: ["" "no active channel" "chZ " "chX  " "chZ & chX " "chY" "chZ & chY  " "chX & chY " "chZ& chX& chY " "INC_X " "chZ & INC_X  " "chX & INC_X" "chZ& chX & INC_X  " "chY & INC_X   " "chZ  & chY & INC_X " "chX  & chY & INC_X " "chZ& chX  & chY & INC_X " "INC_Y is " " chZ & INC_Y " " chX & INC_Y  " "chZ & chX & INC_Y " " chY & INC_Y  " "chZ & chY & INC_Y " "chX & chY & INC_Y  " " chZ &chX & chY & INC_Y" " INC_X & INC_Y " "chZ &   INC_X & INC_Y" "chX & INC_X & INC_Y  " " chZ & chX &  INC_X & INC_Y  " " chY &  INC_X & INC_Y " "chZ & chY &  INC_X & INC_Y " "chX & chY &  INC_X & INC_Y" "chZ & chX & chY &  INC_X & INC_Y"] -> w441
              tunnel: w440 -> [_ _ w576 w635 w696 w758 w820 w885 w953 w1018 w1080 w1145 w1213 w1281 w1349 w1420 w1494 w1562 w1624 w1688 w1756 w1823 w1891 w1962 w2033 w2102 w2168 w2237 w2308 w2380 w2451 w2525 w2601]
              tunnel: [_ _ w573 w632 w692 w755 w818 w881 w949 w1017 w1077 w1143 w1209 w1277 w1345 w1415 w1489 w1559 w1621 w1685 w1753 w1820 w1888 w1959 w2028 w2098 w2164 w2233 w2307 w2375 w2448 w2519 w2594] -> w410
              tunnel: w437 -> [_ _ w575 w634 w695 w756 w819 w884 w948 w1016 w1078 w1144 w1212 w1280 w1348 w1419 w1493 w1561 w1623 w1687 w1755 w1822 w1890 w1960 w2029 w2101 w2167 w2234 w2304 w2379 w2450 w2523 w2596]
              tunnel: [_ _ w572 _ w691 _ w815 _ w947 _ w1075 _ w1207 _ w1343 _ w1487 _ w1619 _ w1750 _ w1885 _ w2026 _ w2162 _ w2301 _ w2444 _ w2593] -> w453
              tunnel: [_ _ _ w631 w690 _ _ w880 w946 _ _ w1140 w1206 _ _ w1414 w1486 _ _ w1683 w1749 _ _ w1956 w2025 _ _ w2231 w2300 _ _ w2518 w2592] -> w452
              tunnel: [_ _ _ _ _ w754 w814 w879 w945 _ _ _ _ w1276 w1342 w1413 w1485 _ _ _ _ w1818 w1884 w1955 w2024 _ _ _ _ w2374 w2443 w2517 w2591] -> w451
              tunnel: [_ _ _ _ _ _ _ _ _ w1014 w1074 w1139 w1205 w1275 w1341 w1412 w1484 _ _ _ _ _ _ _ _ w2097 w2161 w2230 w2299 w2373 w2442 w2516 w2590] -> w450
              tunnel: [_ _ _ _ _ _ _ _ _ _ _ _ _ _ _ _ _ w1558 w1618 w1682 w1748 w1817 w1883 w1954 w2023 w2096 w2160 w2229 w2298 w2372 w2441 w2515 w2589] -> w449
              tunnel: w439 -> [_ _ w571 w629 w688 w752 w812 w877 w943 w1012 w1072 w1137 w1203 w1273 w1339 w1410 w1482 w1556 w1616 w1680 w1746 w1815 w1881 w1952 w2021 w2094 w2158 w2227 w2296 w2370 w2439 w2513 w2587]
              tunnel: w438 -> [_ _ w570 w630 w689 w753 w813 w878 w944 w1013 w1073 w1138 w1204 w1274 w1340 w1411 w1483 w1557 w1617 w1681 w1747 w1816 w1882 w1953 w2022 w2095 w2159 w2228 w2297 w2371 w2440 w2514 w2588]
              tunnel: w437 -> [_ _ w569 w628 w687 w751 w811 w876 w942 w1011 w1071 w1136 w1202 w1272 w1338 w1409 w1481 w1555 w1615 w1679 w1745 w1814 w1880 w1951 w2020 w2093 w2157 w2226 w2295 w2369 w2438 w2512 w2586]
              tunnel: w436 -> [_ _ w568 w627 w686 w750 w810 w875 w941 w1010 w1070 w1135 w1201 w1271 w1337 w1408 w1480 w1554 w1614 w1678 w1744 w1813 w1879 w1950 w2019 w2092 w2156 w2225 w2294 w2368 w2437 w2511 w2585]
              tunnel: [_ _ w567 _ w685 _ w809 _ w940 _ w1069 _ w1200 _ w1336 _ w1479 _ w1613 _ w1743 _ w1878 _ w2018 _ w2155 _ w2293 _ w2436 _ w2584] -> w448
              tunnel: [_ _ _ w626 w685 _ _ w874 w939 _ _ w1134 w1199 _ _ w1407 w1478 _ _ w1677 w1742 _ _ w1949 w2018 _ _ w2224 w2293 _ _ w2510 w2584] -> w447
              tunnel: [_ _ _ _ _ w749 w808 w873 w938 _ _ _ _ w1270 w1335 w1406 w1477 _ _ _ _ w1812 w1877 w1948 w2018 _ _ _ _ w2367 w2436 w2510 w2584] -> w446
              tunnel: [_ _ _ _ _ _ _ _ _ w1009 w1068 w1133 w1198 w1269 w1334 w1405 w1476 _ _ _ _ _ _ _ _ w2091 w2155 w2224 w2293 w2367 w2436 w2510 w2584] -> w445
              tunnel: [_ _ _ _ _ _ _ _ _ _ _ _ _ _ _ _ _ w1553 w1612 w1677 w1741 w1812 w1876 w1947 w2018 w2091 w2155 w2224 w2293 w2367 w2436 w2510 w2584] -> w443
              tunnel: w427 -> [_ _ w553 w603 w662 w726 w784 w850 w915 w986 w1045 w1110 w1175 w1246 w1311 w1382 w1453 w1530 w1589 w1653 w1718 w1788 w1853 w1924 w1994 w2068 w2132 w2201 w2270 w2344 w2413 w2487 w2561]
              tunnel: [_ _ w543 w602 w661 w725 w785 w849 w914 w985 w1044 w1109 w1174 w1245 w1310 w1381 w1452 w1529 w1588 w1654 w1717 w1789 w1852 w1923 w1995 w2067 w2131 w2200 w2269 w2343 w2412 w2486 w2560] -> w444
              tunnel: w406 -> [_ _ w542 w601 w660 w724 w783 w848 w913 w984 w1043 w1108 w1173 w1244 w1309 w1380 w1451 w1528 w1587 w1652 w1716 w1787 w1851 w1922 w1993 w2066 w2130 w2199 w2268 w2342 w2411 w2485 w2559]
              frame Default {
              }
              frame 0 {
              }
              frame 1 {
                w548 = T14 2 items=["User Home"=0, "User Desktop"=1, "User Documents"=2, "User Application Data"=3, "User Preferences"=4, "User Temporary"=5, "Public Documents"=6, "Public Application Data"=7, "Public Preferences"=8, "Public Cache"=13, "System Core Libraries"=9, "System Installed Libraries"=10, "Application Files"=11, "Boot Volume Root"=12] ("system directory type")
                n258 = Decimate 1D Array(w576) -> (w574:dbl[])
                n259 = Search and Replace String(replace all?=TRUE ("replace all? (F)"), input string=w553, search string="/") -> (result string=w565:string)  [unwired: 5 in, 3 out]
                n260 = Concatenate Strings(w542, "TimeStamp;MeasureCh_Z(g);", "\n") -> (w558:string)
                n261 = for {
                  tunnel: w574 -> [w595] mode=indexing
                  tunnel: [w598] -> w573 mode=indexing
                  tunnel: w575 -> [w597] mode=indexing
                  tunnel: [w595] -> w572 mode=indexing
                  tunnel: w571 -> [w590]
                  tunnel: w570 -> [w589]
                  tunnel: w569 -> [w588] mode=indexing
                  tunnel: w568 -> [w587]
                  tunnel: [w581] -> w567
                  n262 = Join Numbers(hi=w589, lo=w590) -> ((hi.lo)=w592:u32)
                  n263 = To Double Precision Float(number=w588) -> (double precision float=w593:dbl)
                  n264 = Number To Decimal String(number=w597) -> (decimal integer string=w596:string)  [unwired: 1 in]
                  n265 = Number To Fractional String(number=w595, precision (6)=i16 3 ("width (-)")) -> (F-format string=w599:string)  [unwired: 2 in]
                  n266 = Divide(x=w593, y=w587) -> (x/y=w594:dbl)
                  n267 = To Unsigned Quad Integer(1:w592) -> (0:w591:u64)
                  n268 = Build Array(w596, w599) -> (w598:string[])
                  n269 = call "Unix Time to Timestamp.vi"("Fractional Second"=w594, "Unix Time (s)"=w591) -> ("Timestamp"=w582:timestamp)  [unwired: 8 in, 1 out]
                  n270 = Format Date/Time String(seconds (now)=w582, UTC format=TRUE) -> (date/time string=w583:string)  [unwired: 1 in]
                  n271 = Scan From String(format string="%<%x %H:%M:%S%3u>T", input string=w583) -> (output 1=w584:timestamp)  [unwired: 3 in, 3 out]
                  n272 = To Double Precision Float(number=w584) -> (double precision float=w581:dbl)
                }
                n273 = Concatenate Strings(w565, "_" ("string"), "streaming.csv") -> (w566:string)
                n274 = call <vilib>:"Get System Directory.vi"("system directory type"=w548) -> ("system directory"=w559:path)  [unwired: 10 in]
                n275 = Build Path(base path=w559, name or relative path="Logfile") -> (appended path=w560:path)
                n276 = call <vilib>:"Check if File or Folder Exists.vi"("path"=w560) -> ("file or folder exists?"=w561:bool, "dup path"=w562:path)  [unwired: 8 in, 1 out]
                n277 = case shown="False" w561 {
                  tunnel: w562 -> [w579 w580]
                  tunnel: [w578 w580] -> w563
                  frame False {
                    n278 = Create Folder(path (use dialog)=w579) -> (created path=w578:path)  [unwired: 2 in, 2 out]
                  }
                  frame True {
                  }
                }
                n279 = Build Path(base path=w563, name or relative path=w566) -> (appended path=w564:path)
                n280 = Open/Create/Replace File(file path (use dialog)=w564, operation (0:open)=T11."open or create") -> (refnum out=w557:refnum<file>, error out=w555:errorcluster)  [unwired: 4 in, 1 out]
                n281 = Write to Text File(file (use dialog)=w557, text=w558, error in=w555) -> (refnum out=w556:refnum<file>, error out=w554:errorcluster)  [unwired: 1 in, 1 out]
                n282 = Close File(refnum=w556, error in=w554) -> (path=w543:path)  [unwired: 1 out]
              }
              frame 2 {
                w608 = T14 2 items=["User Home"=0, "User Desktop"=1, "User Documents"=2, "User Application Data"=3, "User Preferences"=4, "User Temporary"=5, "Public Documents"=6, "Public Application Data"=7, "Public Preferences"=8, "Public Cache"=13, "System Core Libraries"=9, "System Installed Libraries"=10, "Application Files"=11, "Boot Volume Root"=12] ("system directory type")
                n283 = Decimate 1D Array(w635) -> (w633:dbl[])
                n284 = Search and Replace String(replace all?=TRUE ("replace all? (F)"), input string=w603, search string="/") -> (result string=w624:string)  [unwired: 5 in, 3 out]
                n285 = for {
                  tunnel: w633 -> [w654] mode=indexing
                  tunnel: [w657] -> w632 mode=indexing
                  tunnel: w634 -> [w656] mode=indexing
                  tunnel: [w654] -> w631 mode=indexing
                  tunnel: w630 -> [w649]
                  tunnel: w629 -> [w648]
                  tunnel: w628 -> [w647] mode=indexing
                  tunnel: w627 -> [w646]
                  tunnel: [w640] -> w626
                  n286 = Join Numbers(hi=w649, lo=w648) -> ((hi.lo)=w651:u32)
                  n287 = To Double Precision Float(number=w647) -> (double precision float=w652:dbl)
                  n288 = Number To Decimal String(number=w656) -> (decimal integer string=w655:string)  [unwired: 1 in]
                  n289 = Number To Fractional String(number=w654, precision (6)=i16 3 ("width (-)")) -> (F-format string=w658:string)  [unwired: 2 in]
                  n290 = Divide(x=w652, y=w646) -> (x/y=w653:dbl)
                  n291 = To Unsigned Quad Integer(1:w651) -> (0:w650:u64)
                  n292 = Build Array(w655, w658) -> (w657:string[])
                  n293 = call "Unix Time to Timestamp.vi"("Fractional Second"=w653, "Unix Time (s)"=w650) -> ("Timestamp"=w641:timestamp)  [unwired: 8 in, 1 out]
                  n294 = Format Date/Time String(seconds (now)=w641, UTC format=TRUE) -> (date/time string=w642:string)  [unwired: 1 in]
                  n295 = Scan From String(format string="%<%x %H:%M:%S%3u>T", input string=w642) -> (output 1=w643:timestamp)  [unwired: 3 in, 3 out]
                  n296 = To Double Precision Float(number=w643) -> (double precision float=w640:dbl)
                }
                n297 = Concatenate Strings(w601, "TimeStamp;MeasureCh_X(g);", "\n") -> (w617:string)
                n298 = Concatenate Strings(w624, "_" ("string"), "streaming.csv") -> (w625:string)
                n299 = call <vilib>:"Get System Directory.vi"("system directory type"=w608) -> ("system directory"=w618:path)  [unwired: 10 in]
                n300 = Build Path(base path=w618, name or relative path="Logfile") -> (appended path=w619:path)
                n301 = call <vilib>:"Check if File or Folder Exists.vi"("path"=w619) -> ("file or folder exists?"=w620:bool, "dup path"=w621:path)  [unwired: 8 in, 1 out]
                n302 = case shown="False" w620 {
                  tunnel: w621 -> [w638 w639]
                  tunnel: [w637 w639] -> w622
                  frame False {
                    n303 = Create Folder(path (use dialog)=w638) -> (created path=w637:path)  [unwired: 2 in, 2 out]
                  }
                  frame True {
                  }
                }
                n304 = Build Path(base path=w622, name or relative path=w625) -> (appended path=w623:path)
                n305 = Open/Create/Replace File(file path (use dialog)=w623, operation (0:open)=T11."open or create") -> (refnum out=w616:refnum<file>, error out=w614:errorcluster)  [unwired: 4 in, 1 out]
                n306 = Write to Text File(file (use dialog)=w616, text=w617, error in=w614) -> (refnum out=w615:refnum<file>, error out=w613:errorcluster)  [unwired: 1 in, 1 out]
                n307 = Close File(refnum=w615, error in=w613) -> (path=w602:path)  [unwired: 1 out]
              }
              frame 3 {
                w667 = T14 2 items=["User Home"=0, "User Desktop"=1, "User Documents"=2, "User Application Data"=3, "User Preferences"=4, "User Temporary"=5, "Public Documents"=6, "Public Application Data"=7, "Public Preferences"=8, "Public Cache"=13, "System Core Libraries"=9, "System Installed Libraries"=10, "Application Files"=11, "Boot Volume Root"=12] ("system directory type")
                n308 = Decimate 1D Array(w696) -> (w694:dbl[], w693:dbl[])
                n309 = Search and Replace String(replace all?=TRUE ("replace all? (F)"), input string=w662, search string="/") -> (result string=w683:string)  [unwired: 5 in, 3 out]
                n310 = for {
                  tunnel: w694 -> [w716] mode=indexing
                  tunnel: w693 -> [w715] mode=indexing
                  tunnel: [w719] -> w692 mode=indexing
                  tunnel: w695 -> [w718] mode=indexing
                  tunnel: [w716] -> w691 mode=indexing
                  tunnel: [w715] -> w690 mode=indexing
                  tunnel: w689 -> [w710]
                  tunnel: w688 -> [w709]
                  tunnel: w687 -> [w708] mode=indexing
                  tunnel: w686 -> [w707]
                  tunnel: [w701] -> w685
                  n311 = Join Numbers(hi=w710, lo=w709) -> ((hi.lo)=w712:u32)
                  n312 = To Double Precision Float(number=w708) -> (double precision float=w713:dbl)
                  n313 = Number To Decimal String(number=w718) -> (decimal integer string=w717:string)  [unwired: 1 in]
                  n314 = Number To Fractional String(number=w716, precision (6)=i16 3 ("width (-)")) -> (F-format string=w721:string)  [unwired: 2 in]
                  n315 = Number To Fractional String(number=w715, precision (6)=i16 3 ("width (-)")) -> (F-format string=w720:string)  [unwired: 2 in]
                  n316 = Divide(x=w713, y=w707) -> (x/y=w714:dbl)
                  n317 = Build Array(w717, w721, w720) -> (w719:string[])
                  n318 = To Unsigned Quad Integer(1:w712) -> (0:w711:u64)
                  n319 = call "Unix Time to Timestamp.vi"("Fractional Second"=w714, "Unix Time (s)"=w711) -> ("Timestamp"=w702:timestamp)  [unwired: 8 in, 1 out]
                  n320 = Format Date/Time String(seconds (now)=w702, UTC format=TRUE) -> (date/time string=w703:string)  [unwired: 1 in]
                  n321 = Scan From String(format string="%<%x %H:%M:%S%3u>T", input string=w703) -> (output 1=w704:timestamp)  [unwired: 3 in, 3 out]
                  n322 = To Double Precision Float(number=w704) -> (double precision float=w701:dbl)
                }
                n323 = Concatenate Strings(w660, "TimeStamp;MeasureCh_Z(g);Ch_X(g);", "\n") -> (w676:string)
                n324 = Concatenate Strings(w683, "_" ("string"), "streaming.csv") -> (w684:string)
                n325 = call <vilib>:"Get System Directory.vi"("system directory type"=w667) -> ("system directory"=w677:path)  [unwired: 10 in]
                n326 = Build Path(base path=w677, name or relative path="Logfile") -> (appended path=w678:path)
                n327 = call <vilib>:"Check if File or Folder Exists.vi"("path"=w678) -> ("file or folder exists?"=w679:bool, "dup path"=w680:path)  [unwired: 8 in, 1 out]
                n328 = case shown="False" w679 {
                  tunnel: w680 -> [w699 w700]
                  tunnel: [w698 w700] -> w681
                  frame False {
                    n329 = Create Folder(path (use dialog)=w699) -> (created path=w698:path)  [unwired: 2 in, 2 out]
                  }
                  frame True {
                  }
                }
                n330 = Build Path(base path=w681, name or relative path=w684) -> (appended path=w682:path)
                n331 = Open/Create/Replace File(file path (use dialog)=w682, operation (0:open)=T11."open or create") -> (refnum out=w675:refnum<file>, error out=w673:errorcluster)  [unwired: 4 in, 1 out]
                n332 = Write to Text File(file (use dialog)=w675, text=w676, error in=w673) -> (refnum out=w674:refnum<file>, error out=w672:errorcluster)  [unwired: 1 in, 1 out]
                n333 = Close File(refnum=w674, error in=w672) -> (path=w661:path)  [unwired: 1 out]
              }
              frame 4 {
                w731 = T14 2 items=["User Home"=0, "User Desktop"=1, "User Documents"=2, "User Application Data"=3, "User Preferences"=4, "User Temporary"=5, "Public Documents"=6, "Public Application Data"=7, "Public Preferences"=8, "Public Cache"=13, "System Core Libraries"=9, "System Installed Libraries"=10, "Application Files"=11, "Boot Volume Root"=12] ("system directory type")
                n334 = Decimate 1D Array(w758) -> (w757:dbl[])
                n335 = Search and Replace String(replace all?=TRUE ("replace all? (F)"), input string=w726, search string="/") -> (result string=w747:string)  [unwired: 5 in, 3 out]
                n336 = for {
                  tunnel: w757 -> [w777] mode=indexing
                  tunnel: [w780] -> w755 mode=indexing
                  tunnel: w756 -> [w779] mode=indexing
                  tunnel: [w777] -> w754 mode=indexing
                  tunnel: w753 -> [w772]
                  tunnel: w752 -> [w769]
                  tunnel: w751 -> [w770] mode=indexing
                  tunnel: w750 -> [w771]
                  tunnel: [w763] -> w749
                  n337 = Join Numbers(hi=w772, lo=w769) -> ((hi.lo)=w774:u32)
